vi "Format Signed Identifier.vi"(11 "Signed identifier":T1) -> (3 "Signed identifier string":string)   [LabVIEW 2015, in "NI_Azure_Queue.lvlib"]
uses:
  NI_Azure_Queue.lvlib
  Signed Identifier.ctl
  Access Policy.ctl
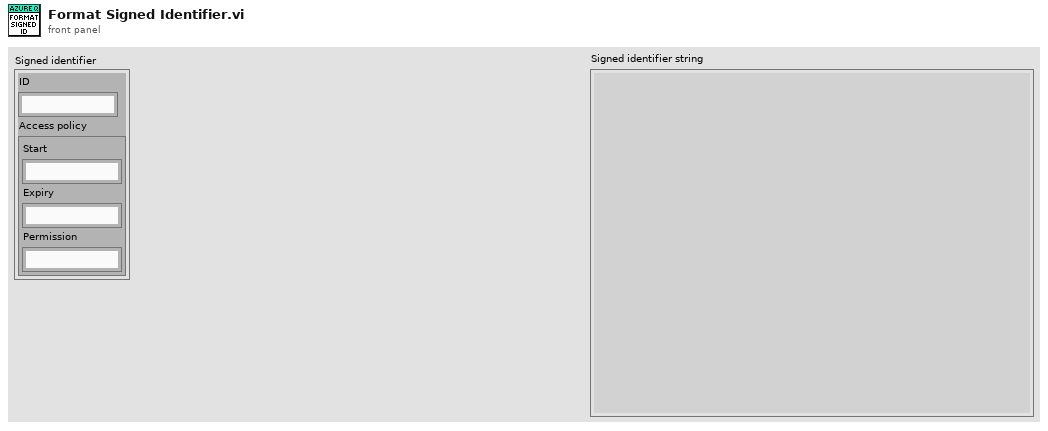
[diagram p1: front panel]
types:
  T1 = typedef "NI_Azure_Queue.lvlib/Signed Identifier.ctl" = cluster{"ID":string, "Access policy":T2}
  T2 = typedef "NI_Azure_Queue.lvlib/Access Policy.ctl" = cluster{"Start":string, "Expiry":string, "Permission":string}
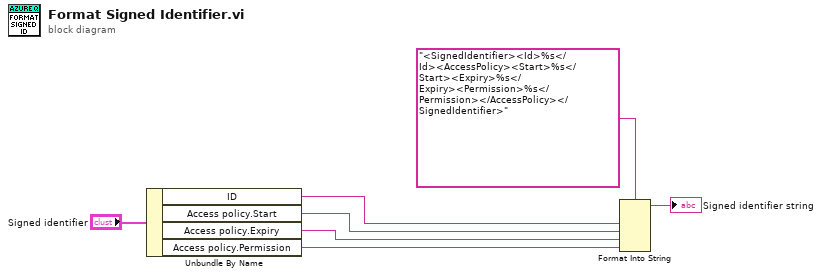
[diagram p0: block diagram]
diagram:
  n1 = Unbundle By Name("Signed identifier") -> ("ID"=w4:string, "Access policy.Start"=w3:string, "Access policy.Expiry"=w2:string, "Access policy.Permission"=w1:string)
  n2 = Format Into String(format string="<SignedIdentifier><Id>%s</Id><AccessPolicy><Start>%s</Start><Expiry>%s</Expiry><Permission>%s</Permission></AccessPolicy></SignedIdentifier>", w4, w3, w2, w1) -> (resulting string=→"Signed identifier string":string)  [unwired: 2 in, 1 out]
